vi "CMI Sync V3 Panel.vi"(8 "error in":errorcluster, 11 "session in":T1={"VISA"="", "baud rate [bd/s]"=115200, "source"=enum."Auto", "hv range"=enum."1kV", "fsrc is fixed"=FALSE, "fsrc [Hz]"=10000000.0, "freq integ [s]"=1.0, "freq filter"=5, "trig level"=enum."TTL 5V", "chn1 mode"=enum."Source divider", "chn1 level"=enum."Positive 5V", "chn2 mode"=enum."Source divider", "chn2 level"=enum."Positive 5V", "chn2 div"=1, "chn3 mode"=enum."Chn 1 Active", "chn3 level"=enum."Positive 5V"} {"chn2 div" min=1 max=100000000 step=1; "fsrc [Hz]" format="%_8p"}) -> (0 "error out":errorcluster, 3 "session out":T1={"VISA"="", "baud rate [bd/s]"=115200, "source"=enum."Auto", "hv range"=enum."1kV", "fsrc is fixed"=FALSE, "fsrc [Hz]"=10000000.0, "freq integ [s]"=1.0, "freq filter"=5, "trig level"=enum."TTL 5V", "chn1 mode"=enum."Source divider", "chn1 level"=enum."Positive 5V", "chn2 mode"=enum."Source divider", "chn2 level"=enum."Positive 5V", "chn2 div"=1, "chn3 mode"=enum."Chn 1 Active", "chn3 level"=enum."Positive 5V"} {"chn2 div" min=1 max=100000000 step=1; "fsrc [Hz]" format="%_8p"})   [LabVIEW 2020, in "AWG.lvlib" / "CMI Sync Unit V3.lvlib"]
doc: "Configuration panel of CMI Sync Unit V3. Sets the basic setup that is not intended to be changed after opening the device."
uses:
  CMI Sync Unit V3.lvlib
  Configure/CMI Sync V3 Reference Clock Source.ctl
  Configure/CMI Sync V3 HV input Range.ctl
  Configure/CMI Sync V3 Channel 1 Mode.ctl
  Configure/CMI Sync V3 Trigger Input Level.ctl
  Configure/CMI Sync V3 Channel 2 Mode.ctl
  Configure/CMI Sync V3 Channel Output Levels.ctl
  Configure/CMI Sync V3 Channel 3 Mode.ctl
  CMI Sync V3 session.ctl
  varilib/SGUI Assign References Mode.ctl
  varilib/SGUI Assign Multiple Strings With Tags By Label.vi
  varilib/SGUI Set Single Real By Label.vi
  varilib/varilib.lvlib
panel:
  out "err string":string caption="Error"
  out "meas freq":dbl caption="Source frequency [Hz]" format="%0_8p"
  out "idn string":string caption="Device identification"
  in  "btn check":bool
  in  "btn ok":bool caption="OK"
  in  "fsrc":dbl=10000000.0 caption="Source frequency [Hz]" format="%_8p"
  in  "fsrc fixed":bool caption="Define source freq. here:"
  in  "chn3 level":T6=enum."Positive 5V" caption="Channel 3 output levels"
  in  "chn3 mode":T8 caption="Channel 3 mode"
  in  "chn2 level":T6=enum."Positive 5V" caption="Channel 2 output levels"
  in  "chn1 level":T6=enum."Positive 5V" caption="Channel 1 output levels"
  in  "chn2 div":i32=1 caption="Channel 2 divisor" min=1 max=100000000 step=1
  in  "chn2 mode":T7 caption="Channel 2 mode"
  in  "trig level":T4=enum."TTL 5V" caption="Trigger input logic"
  in  "freq filter":i32=5 caption="Counter filtering periods"
  in  "freq integ":dbl=1.0 caption="Counter integration [s]"
  in  "chn1 mode":T5 caption="Channel 1 mode"
  in  "hv range":T3=enum."1kV" caption="HV input range"
  in  "VISA address":refnum<visa-resource-name>
  in  "source":T2 caption="Clock source"
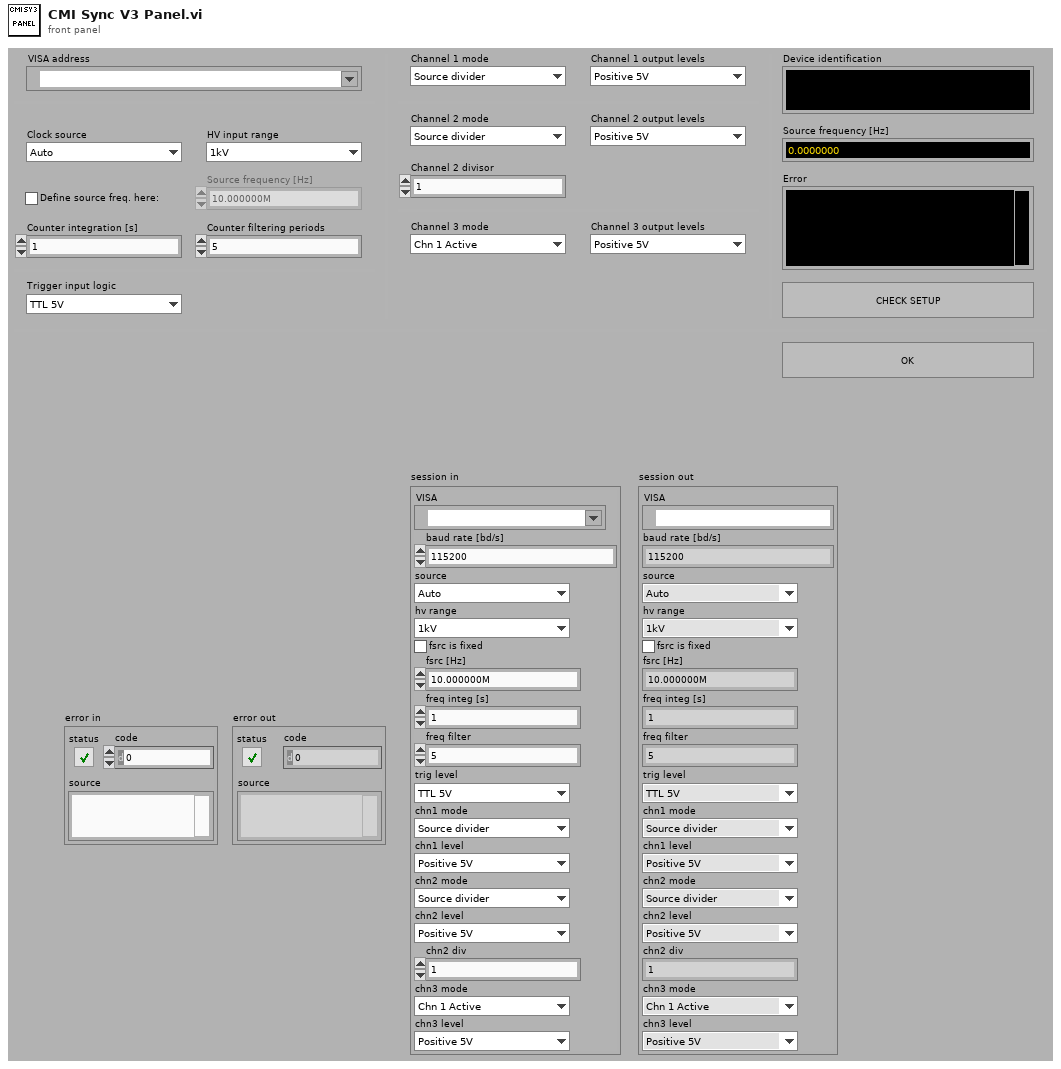
[diagram p1: front panel]
types:
  T1 = typedef "AWG.lvlib/CMI Sync Unit V3.lvlib/CMI Sync V3 session.ctl" = cluster{"VISA":refnum<visa-resource-name>, "baud rate [bd/s]":i32, "source":T2, "hv range":T3, "fsrc is fixed":bool, "fsrc [Hz]":dbl, "freq integ [s]":dbl, "freq filter":i32, "trig level":T4, "chn1 mode":T5, "chn1 level":T6, "chn2 mode":T7, "chn2 level":T6, "chn2 div":i32, "chn3 mode":T8, "chn3 level":T6}
  T2 = typedef "AWG.lvlib/CMI Sync Unit V3.lvlib/CMI Sync V3 Reference Clock Source.ctl" = enum16{"Auto", "Internal", "Logic", "Sine", "HV"}
  T3 = typedef "AWG.lvlib/CMI Sync Unit V3.lvlib/CMI Sync V3 HV input Range.ctl" = enum16{"10V", "60V", "250V", "1kV"}
  T4 = typedef "AWG.lvlib/CMI Sync Unit V3.lvlib/CMI Sync V3 Trigger Input Level.ctl" = enum16{"LVCMOS 3V3", "TTL 5V"}
  T5 = typedef "AWG.lvlib/CMI Sync Unit V3.lvlib/CMI Sync V3 Channel 1 Mode.ctl" = enum16{"Source divider", "DDS absolute", "DDS ratio", "DDS ratio M/N"}
  T6 = typedef "AWG.lvlib/CMI Sync Unit V3.lvlib/CMI Sync V3 Channel Output Levels.ctl" = enum16{"Positive 3V3", "Negative 3V3", "Positive 5V", "Negative 5V"}
  T7 = typedef "AWG.lvlib/CMI Sync Unit V3.lvlib/CMI Sync V3 Channel 2 Mode.ctl" = enum16{"Source divider", "Chn 1 divide"}
  T8 = typedef "AWG.lvlib/CMI Sync Unit V3.lvlib/CMI Sync V3 Channel 3 Mode.ctl" = enum16{"Chn 1 Active", "Chn 2 Active", "Chn 1 Trigger", "Chn 2 Trigger", "Gate", "PPS", "10MHz"}
  T9 = typedef "varilib.lvlib/SGUI Assign References Mode.ctl" = enum16{"Add to stack", "Overwrite", "Release last", "Release ID"}
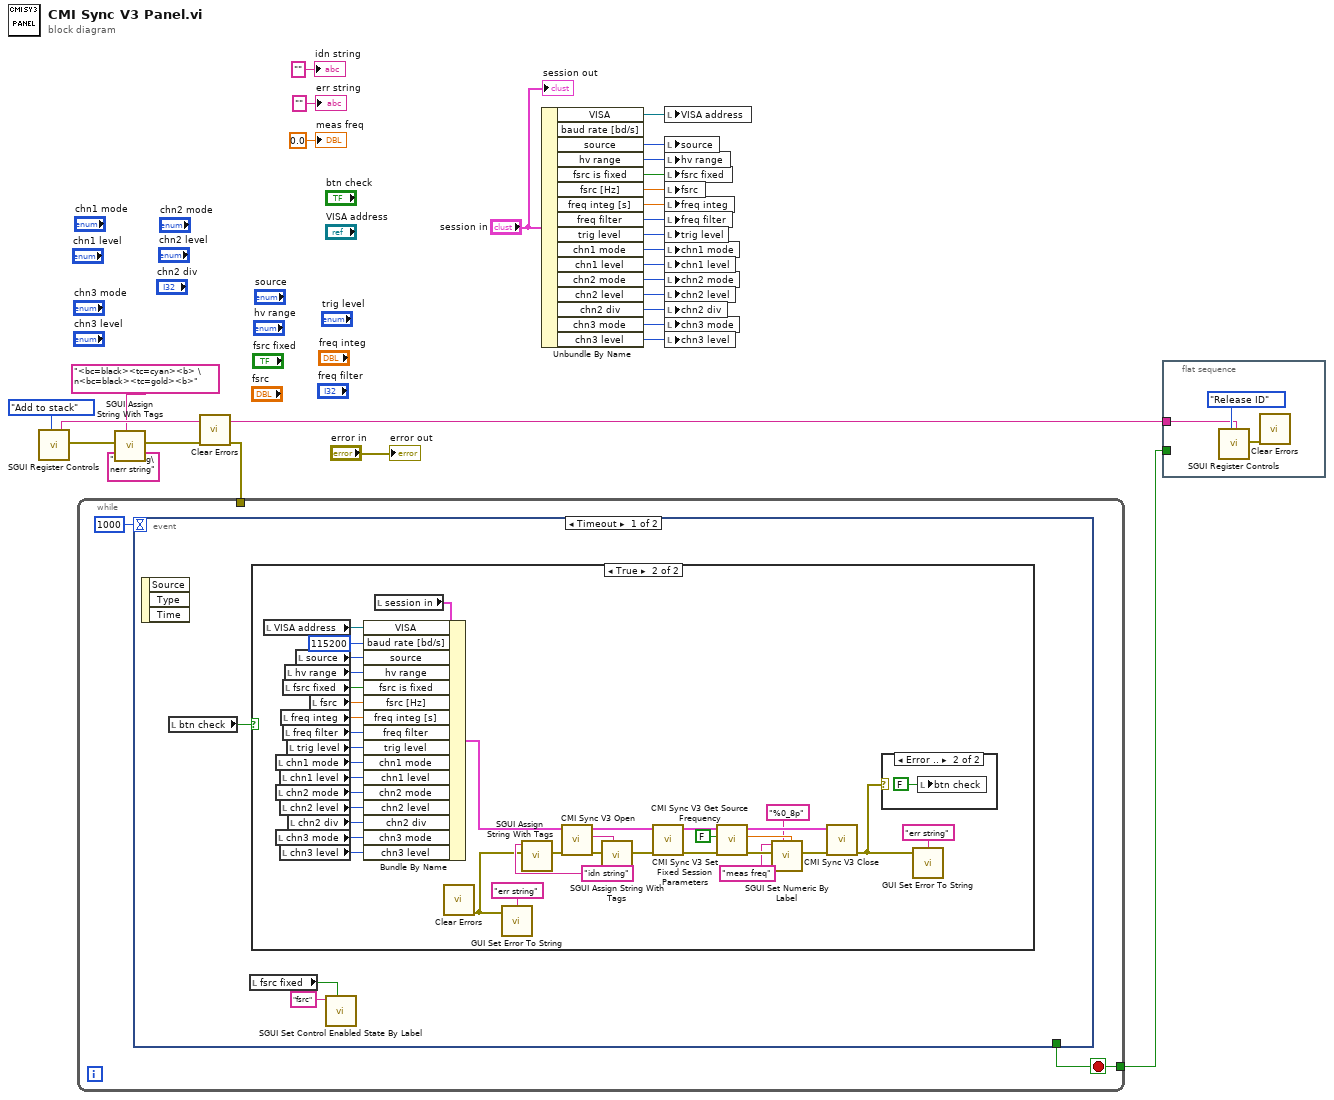
[diagram p0: block diagram]
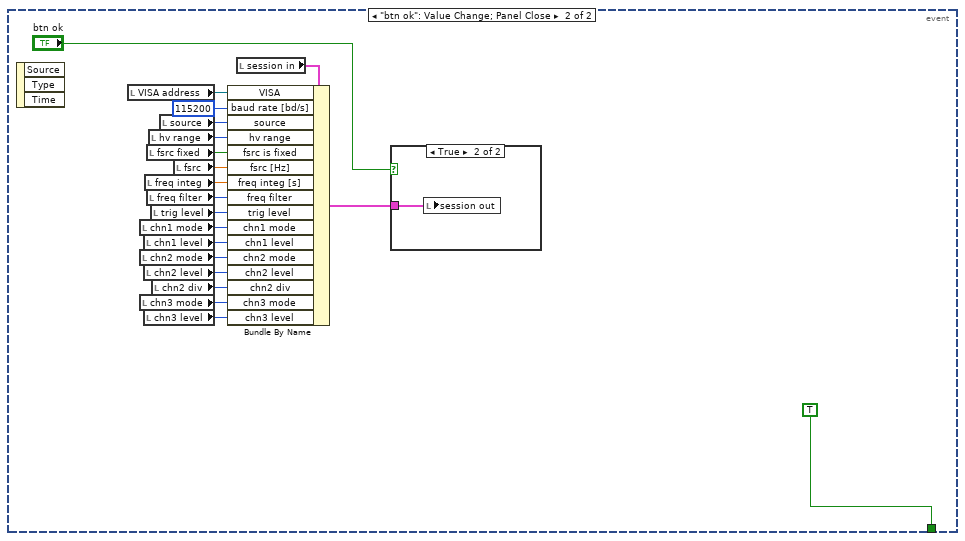
[diagram p4: hidden frame]
diagram:
  n1 = call "SGUI Register Controls.vi"("register mode (overwrite)"=SGUI_Assign_References_Mode."Add to stack") -> ("assigned ID"=w24:string, "error out"=w21:errorcluster)  [unwired: 16 in, 1 out]
  n2 = call-poly "SGUI Assign String With Tags.vi"("error in"=w21, "label(s) (empty)"="idn string\nerr string" ("control label (none)"), "string (empty)"="<bc=black><tc=cyan><b> \n<bc=black><tc=gold><b>" ("control label (none)")) -> ("error out"=w20:errorcluster)  [unwired: 7 in, 1 out]
  n3 = call <vilib>:"Clear Errors.vi"("error in (no error)"=w20) -> ("error out"=w22:errorcluster)  [unwired: 5 in, 1 out]
  n4 = while {
    tunnel: [w30] -> w23
    tunnel: w22 -> [_]
    stop <- w30 stop-if-true
    n5 = event shown="[0] Timeout" {
      selector: _ -> [_ _]
      dyn-events: _ -> [_ _]
      timeout: 1000 -> [_ _]
      tunnel: [_ TRUE] -> w30
      event Timeout {
        n6 = event-data() -> ()  [unwired: 1 in, 3 out]
        n7 = local read "btn check"() -> (w33:bool)
        n8 = local read "fsrc fixed"() -> (w32:bool)
        n9 = case shown="True" w33 {
          frame False {
          }
          frame True {
            w36 = "idn string" ("control label (none)")
            n10 = local read "VISA address"() -> (w70:refnum<visa-resource-name>)
            n11 = local read "chn1 mode"() -> (w62:T5)
            n12 = local read "chn2 mode"() -> (w60:T7)
            n13 = local read "chn3 mode"() -> (w57:T8)
            n14 = local read "chn1 level"() -> (w61:T6)
            n15 = local read "chn2 level"() -> (w59:T6)
            n16 = local read "chn3 level"() -> (w56:T6)
            n17 = local read "freq integ"() -> (w65:dbl)
            n18 = local read "fsrc fixed"() -> (w67:bool)
            n19 = local read "freq filter"() -> (w64:i32)
            n20 = local read "hv range"() -> (w68:T3)
            n21 = local read "trig level"() -> (w63:T4)
            n22 = local read "chn2 div"() -> (w58:i32)
            n23 = local read "source"() -> (w69:T2)
            n24 = local read "fsrc"() -> (w66:dbl)
            n25 = local read "session in"() -> (w38:T1)
            n26 = Bundle By Name(cluster=w38, "VISA"=w70, "baud rate [bd/s]"=115200, "source"=w69, "hv range"=w68, "fsrc is fixed"=w67, "fsrc [Hz]"=w66, "freq integ [s]"=w65, "freq filter"=w64, "trig level"=w63, "chn1 mode"=w62, "chn1 level"=w61, "chn2 mode"=w60, "chn2 level"=w59, "chn2 div"=w58, "chn3 mode"=w57, "chn3 level"=w56) -> (w54:T1)
            n27 = call <vilib>:"Clear Errors.vi"() -> ("error out"=w34:errorcluster)  [unwired: 6 in, 1 out]
            n28 = call "GUI Set Error To String.vi"("error in (no error)"=w34, "label(s) (status)"="err string") -> ()  [unwired: 3 in]
            n29 = call-poly "SGUI Assign String With Tags.vi"("error in"=w34, "label(s) (empty)"=w36) -> ("error out"=w37:errorcluster)  [unwired: 8 in, 1 out]
            n30 = call "CMI Sync V3 Open.vi"("error in"=w37, "session in"=w54) -> ("error out"=w47:errorcluster, "identification string"=w45:string, "session out"=w53:T1)  [unwired: 7 in]
            n31 = call-poly "SGUI Assign String With Tags.vi"("error in"=w47, "label(s) (empty)"=w36, "string (empty)"=w45) -> ("error out"=w46:errorcluster)  [unwired: 7 in, 1 out]
            n32 = call "CMI Sync V3 Set Fixed Session Parameters.vi"("error in"=w46, "session in"=w53) -> ("error out"=w52:errorcluster, "session out"=w51:T1)  [unwired: 8 in]
            n33 = call "CMI Sync V3 Get Source Frequency.vi"("error in"=w52, "Wait for update before? (false)"=FALSE, "session in"=w51) -> ("error out"=w44:errorcluster, "source frequency [Hz]"=w42:dbl, "session out"=w50:T1)  [unwired: 6 in]
            n34 = call-poly "SGUI Set Numeric By Label.vi"("error in"=w44, "label (empty)"="meas freq", "format (empty)"="%0_8p", "value (none)"=w42) -> ("error out"=w43:errorcluster)  [unwired: 6 in, 1 out]
            n35 = call "CMI Sync V3 Close.vi"("error in"=w43, "session in"=w50) -> ("error out"=w48:errorcluster)  [unwired: 8 in, 1 out]
            n36 = case shown="Error .." w48 {
              frame No Error {
              }
              frame Error {
                n37 = local write "btn check"(FALSE ("btn check")) -> ()
              }
            }
            n38 = call "GUI Set Error To String.vi"("error in (no error)"=w48, "label(s) (status)"="err string") -> ()  [unwired: 3 in]
          }
        }
        n39 = call "SGUI Set Control Enabled State By Label.vi"("labels (empty)"="fsrc", "Enabled? (False)"=w32) -> ()  [unwired: 8 in, 2 out]
      }
      event "btn ok": Value Change; Panel Close {
        n40 = event-data() -> ()  [unwired: 1 in, 3 out]
        n41 = local read "VISA address"() -> (w91:refnum<visa-resource-name>)
        n42 = local read "chn1 mode"() -> (w82:T5)
        n43 = local read "chn2 mode"() -> (w80:T7)
        n44 = local read "chn3 mode"() -> (w77:T8)
        n45 = local read "chn1 level"() -> (w81:T6)
        n46 = local read "chn2 level"() -> (w79:T6)
        n47 = local read "chn3 level"() -> (w76:T6)
        n48 = local read "freq integ"() -> (w85:dbl)
        n49 = local read "fsrc fixed"() -> (w87:bool)
        n50 = local read "freq filter"() -> (w84:i32)
        n51 = local read "hv range"() -> (w88:T3)
        n52 = local read "trig level"() -> (w83:T4)
        n53 = local read "chn2 div"() -> (w78:i32)
        n54 = local read "source"() -> (w89:T2)
        n55 = local read "fsrc"() -> (w86:dbl)
        n56 = local read "session in"() -> (w74:T1)
        n57 = Bundle By Name(cluster=w74, "VISA"=w91, "baud rate [bd/s]"=115200, "source"=w89, "hv range"=w88, "fsrc is fixed"=w87, "fsrc [Hz]"=w86, "freq integ [s]"=w85, "freq filter"=w84, "trig level"=w83, "chn1 mode"=w82, "chn1 level"=w81, "chn2 mode"=w80, "chn2 level"=w79, "chn2 div"=w78, "chn3 mode"=w77, "chn3 level"=w76) -> (w73:T1)
        n58 = case shown="True" "btn ok" {
          tunnel: w73 -> [_ w92]
          frame False {
          }
          frame True {
            n59 = local write "session out"(w92) -> ()
          }
        }
      }
    }
  }
  n60 = Unbundle By Name("session in") -> ("VISA"=w16:refnum<visa-resource-name>, "source"=w15:T2, "hv range"=w14:T3, "fsrc is fixed"=w13:bool, "fsrc [Hz]"=w12:dbl, "freq integ [s]"=w11:dbl, "freq filter"=w10:i32, "trig level"=w9:T4, "chn1 mode"=w8:T5, "chn1 level"=w7:T6, "chn2 mode"=w6:T7, "chn2 level"=w5:T6, "chn2 div"=w4:i32, "chn3 mode"=w3:T8, "chn3 level"=w2:T6)  [unwired: 1 out]
  n61 = local write "VISA address"(w16) -> ()
  n62 = local write "source"(w15) -> ()
  n63 = local write "hv range"(w14) -> ()
  n64 = local write "fsrc fixed"(w13) -> ()
  n65 = local write "fsrc"(w12) -> ()
  n66 = local write "freq integ"(w11) -> ()
  n67 = local write "freq filter"(w10) -> ()
  n68 = local write "trig level"(w9) -> ()
  n69 = local write "chn1 mode"(w8) -> ()
  n70 = local write "chn1 level"(w7) -> ()
  n71 = local write "chn2 mode"(w6) -> ()
  n72 = local write "chn2 level"(w5) -> ()
  n73 = local write "chn2 div"(w4) -> ()
  n74 = local write "chn3 mode"(w3) -> ()
  n75 = local write "chn3 level"(w2) -> ()
  n76 = flat-sequence {
    tunnel: w24 -> [w94]
    tunnel: w23 -> [_]
    frame #0 {
      n77 = call "SGUI Register Controls.vi"("register mode (overwrite)"=SGUI_Assign_References_Mode."Release ID", "controls ID (empty)"=w94) -> ("error out"=w93:errorcluster)  [unwired: 15 in, 2 out]
      n78 = call <vilib>:"Clear Errors.vi"("error in (no error)"=w93) -> ()  [unwired: 5 in, 2 out]
    }
  }
  "idn string" <- "" ("idn string")
  "meas freq" <- 0.0 ("meas freq")
  "err string" <- "" ("err string")
  "session out" <- "session in"
  "error out" <- "error in"
